vi "231107_Nikon_Control.vi"() -> ()   [LabVIEW 2014]
panel:
  in  "Cluster commandes":T1={"Dia lamp"=TRUE, "Dia lamp intensity"=1689.1304347826087, "Objective"=2, "Light path"=2, "Z pos (µm)"=335593} {"Z pos (µm)" min=0 max=990000 step=100 scale=0.0..990000.0; "Light path" items=["1- Eyepiece"=1, "2- Right"=2, "3- Left + Eyepiece"=3, "4- Left"=4]; "Objective" items=["1- Target"=1, "2- PLAN APO 100X 1,45 Oil"=2, "3- Empty"=3, "4- Empty"=4, "5- Empty"=5, "6- Empty"=6]; "Dia lamp intensity" scale=0.0..2100.0}
  out "Cluster µscope":T2
  in  "stop":bool
  in  "NikonTi2AxLib.INikonTi2AxMicroscope":refnum<k7>
  out "error out":errorcluster={"status"=TRUE, "code"=-9, "source"="Exception occured in Nikon.Ti2.Microscope.1: Failed in 231026_NikonTi2_Indicators_v2.vi"} caption="sortie d'erreur"
  in  "error in":errorcluster caption="entrée d'erreur"
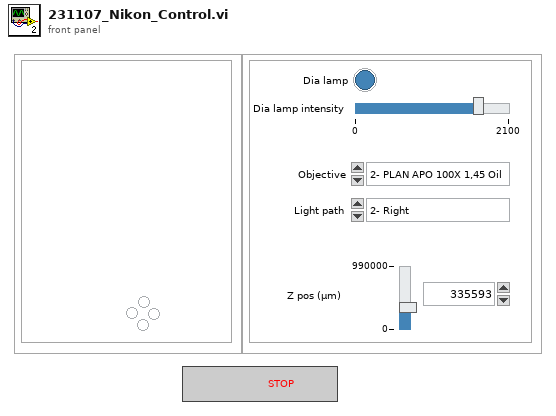
[diagram p1: front panel]
types:
  T1 = cluster{"Dia lamp":bool, "Dia lamp intensity":dbl, "Objective":i32, "Light path":u32, "Z pos (µm)":i32}
  T2 = cluster{"Eyepiece":bool, "Right":bool, "Left + Eyepiece":bool, "Left":bool}
  T3 = cluster{"iNOSEPIECE":i32, "iLIGHTPATH":i32, "iDIA_LAMP_Switch":i32, "iDIA_LAMP_Pos":i32, "iZPOSITION":i32, "iPFS_SWITCH":i32, "iPFS_STATUS":i32, "iPFS_OFFSET":i32}
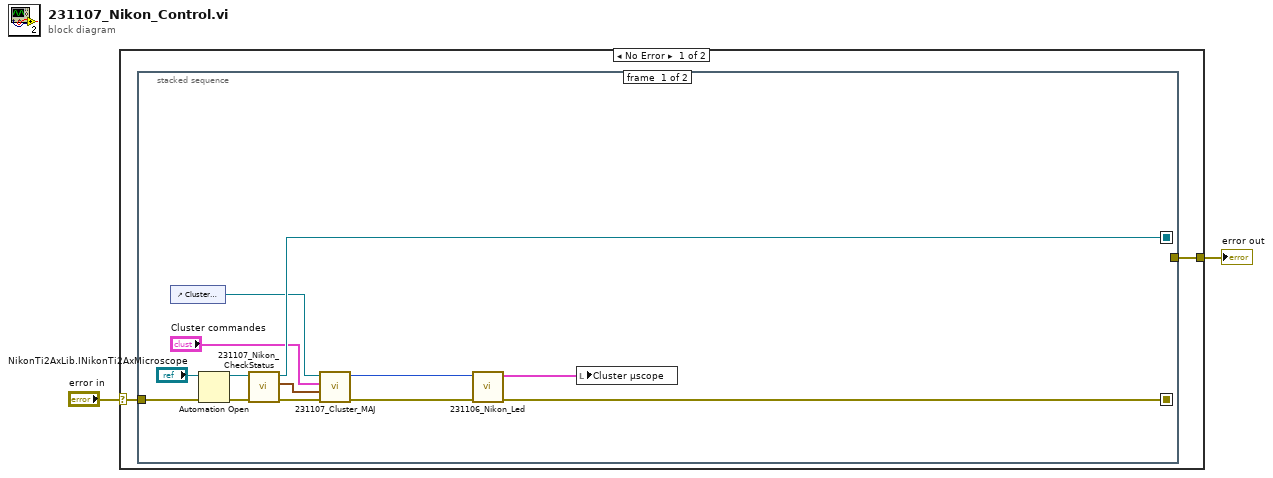
[diagram p0: block diagram]
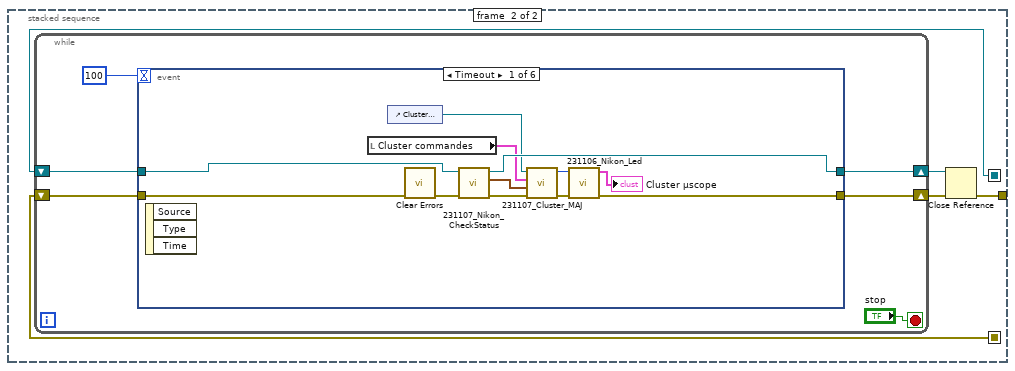
[diagram p2: hidden frame]
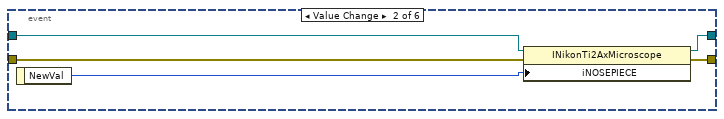
[diagram p3: hidden frame]
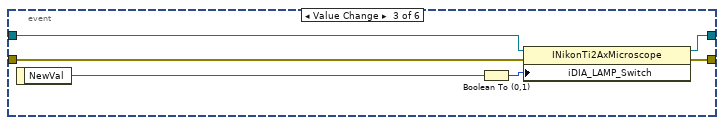
[diagram p4: hidden frame]
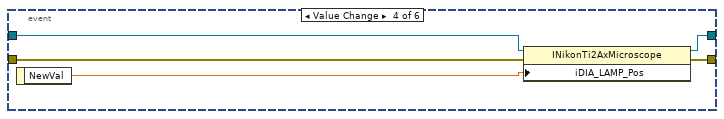
[diagram p5: hidden frame]
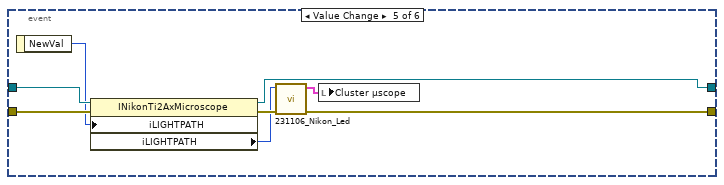
[diagram p6: hidden frame]
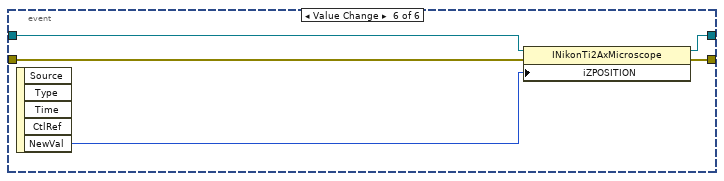
[diagram p7: hidden frame]
diagram:
  n1 = case shown="No Error" "error in" {
    selector: "error in" -> [w4 w70]
    tunnel: [w3 w70] -> w1
    frame No Error {
      n2 = stacked-sequence {
        seq-local: [w13 _] -> [_ w22]
        seq-local: [w6 _] -> [_ w18]
        tunnel: w4 -> [w14 _]
        tunnel: [_ w19] -> w3
        frame #0 {
          n3 = control-ref of="Cluster commandes"() -> (w5:refnum<vi>)
          n4 = Automation Open(error in (no error)=w14, Automation Refnum="NikonTi2AxLib.INikonTi2AxMicroscope") -> (Automation Refnum=w16:refnum<k7>, error out=w15:errorcluster)  [unwired: 2 in]
          n5 = call "231107_Nikon_CheckStatus.vi"("error in"=w15, "NikonTi2AxLib.INikonTi2AxMicroscope"=w16) -> ("error out"=w8:errorcluster, "Nikon status cluster"=w12:T3, "reference out"=w13:refnum<k7>)  [unwired: 7 in]
          n6 = call "231107_Cluster_MAJ.vi"("error in (no error)"=w8, "Nikon status cluster"=w12, 10:"Cluster commandes"="Cluster commandes", 11:"Cluster commandes"=w5) -> ("error out"=w7:errorcluster, "iLIGHTPATH"=w9:i32)  [unwired: 6 in]
          n7 = call "231106_Nikon_Led.vi"("error in"=w7, "Light path"=w9) -> ("error out"=w6:errorcluster, "Cluster µscope"=w11:T2)  [unwired: 8 in]
          n8 = local write "Cluster µscope"(w11) -> ()
        }
        frame #1 {
          n9 = while {
            shift-right: [w23] -> w20
            shift-left: w18 -> [w28]
            shift-right: [w24] -> w21
            shift-left: w22 -> [w25]
            stop <- "stop" stop-if-true
            n10 = event shown="[0] Timeout" {
              selector: _ -> [_ _ _ _ _ _]
              dyn-events: _ -> [_ _ _ _ _ _]
              timeout: 100 -> [_ _ _ _ _ _]
              tunnel: [w29 w42 w48 w53 w61 w68] -> w23
              tunnel: w28 -> [w31 w44 w50 w55 w62 w66]
              tunnel: w25 -> [w40 w45 w51 w56 w63 w67]
              tunnel: [w39 w43 w49 w54 w64 w69] -> w24
              event Timeout {
                n11 = event-data() -> ()  [unwired: 1 in, 3 out]
                n12 = local read "Cluster commandes"() -> (w33:T1)
                n13 = control-ref of="Cluster commandes"() -> (w32:refnum<vi>)
                n14 = call <vilib>:"Clear Errors.vi"("error in (no error)"=w31) -> ("error out"=w30:errorcluster)  [unwired: 5 in, 1 out]
                n15 = call "231107_Nikon_CheckStatus.vi"("error in"=w30, "NikonTi2AxLib.INikonTi2AxMicroscope"=w40) -> ("error out"=w36:errorcluster, "Nikon status cluster"=w37:T3, "reference out"=w39:refnum<k7>)  [unwired: 7 in]
                n16 = call "231107_Cluster_MAJ.vi"("error in (no error)"=w36, "Nikon status cluster"=w37, 10:"Cluster commandes"=w33, 11:"Cluster commandes"=w32) -> ("error out"=w35:errorcluster, "iLIGHTPATH"=w34:i32)  [unwired: 6 in]
                n17 = call "231106_Nikon_Led.vi"("error in"=w35, "Light path"=w34) -> ("error out"=w29:errorcluster, "Cluster µscope"=→"Cluster µscope":T2)  [unwired: 8 in]
              }
              event "Cluster commandes.Objective": Value Change {
                n18 = event-data() -> ("NewVal"=w41:i32)  [unwired: 1 in]
                n19 = property class="INikonTi2AxMicroscope"(reference=w45, error in=w44, "iNOSEPIECE"=w41) -> (reference out=w43:refnum<k7>, error out=w42:errorcluster)
              }
              event "Cluster commandes.Dia lamp": Value Change {
                n20 = event-data() -> ("NewVal"=w47:bool)  [unwired: 1 in]
                n21 = Boolean To (0,1)(Boolean=w47) -> (0, 1=w46:i16)
                n22 = property class="INikonTi2AxMicroscope"(reference=w51, error in=w50, "iDIA_LAMP_Switch"=w46) -> (reference out=w49:refnum<k7>, error out=w48:errorcluster)
              }
              event "Cluster commandes.Dia lamp intensity": Value Change {
                n23 = event-data() -> ("NewVal"=w52:dbl)  [unwired: 1 in]
                n24 = property class="INikonTi2AxMicroscope"(reference=w56, error in=w55, "iDIA_LAMP_Pos"=w52) -> (reference out=w54:refnum<k7>, error out=w53:errorcluster)
              }
              event "Cluster commandes.Light path": Value Change {
                n25 = event-data() -> ("NewVal"=w58:u32)  [unwired: 1 in]
                n26 = property class="INikonTi2AxMicroscope"(reference=w63, error in=w62, "iLIGHTPATH"=w58) -> (reference out=w64:refnum<k7>, error out=w60:errorcluster, "iLIGHTPATH"=w59:i32)
                n27 = call "231106_Nikon_Led.vi"("error in"=w60, "Light path"=w59) -> ("error out"=w61:errorcluster, "Cluster µscope"=w57:T2)  [unwired: 8 in]
                n28 = local write "Cluster µscope"(w57) -> ()
              }
              event "Cluster commandes.Z pos (µm)": Value Change {
                n29 = event-data() -> ("NewVal"=w65:i32)  [unwired: 1 in, 4 out]
                n30 = property class="INikonTi2AxMicroscope"(reference=w67, error in=w66, "iZPOSITION"=w65) -> (reference out=w69:refnum<k7>, error out=w68:errorcluster)
              }
            }
          }
          n31 = Close Reference(reference=w21, error in (no error)=w20) -> (error out=w19:errorcluster)
        }
      }
    }
    frame Error {
    }
  }
  "error out" <- w1
